vi "CloseConnection.vi"(8 "error in (no error)":errorcluster, 11 "II2COUSB in":refnum<class "II2COUSB.lvclass">) -> (0 "error out":errorcluster, 1 "Status":string, 3 "II2COUSB out":refnum<class "II2COUSB.lvclass">)   [LabVIEW 2020, in "II2COUSB.lvlib" / "II2COUSB.lvclass"]
doc: "Close connection"
uses:
  II2COUSB.lvclass
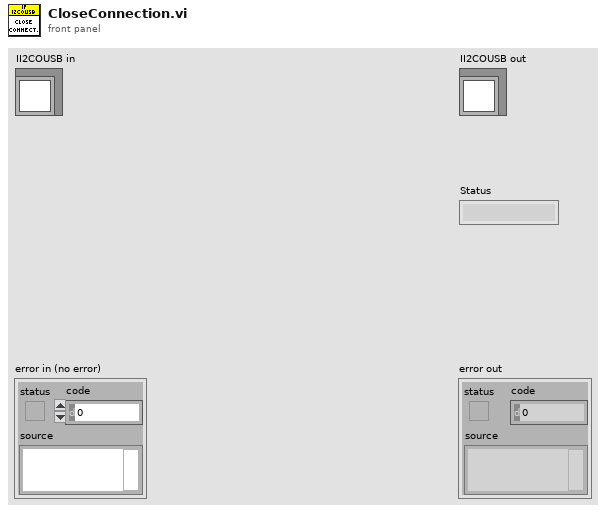
[diagram p1: front panel]
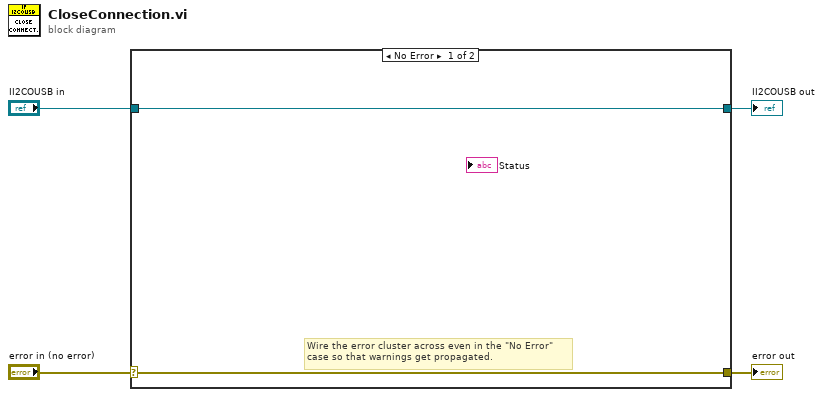
[diagram p0: block diagram]
diagram:
  n1 = case shown="No Error" "error in (no error)" {
    selector: "error in (no error)" -> [w5 w8]
    tunnel: [w5 w8] -> w3
    tunnel: [w6 w7] -> w1
    tunnel: "II2COUSB in" -> [w6 w7]
    frame No Error {
      # "Wire the error cluster across even in the \"No Error\"\ncase so that warnings get propagated."
    }
    frame Error {
    }
  }
  "error out" <- w3
  "II2COUSB out" <- w1
